vi "test Nested-Caller Two Last Acks.vi"(8 "error in (no error)":errorcluster, 11 "TestCase in":refnum<class "Test TCP Nested-Caller Two Last Acks.lvclass">) -> (0 "error out":errorcluster, 3 "TestCase out":refnum<class "Test TCP Nested-Caller Two Last Acks.lvclass">)   [LabVIEW 2020, in "Test TCP Nested-Caller Two Last Acks.lvclass"]
uses:
  Test TCP Nested-Caller Two Last Acks.lvclass
  <vilib>/addons/_JKI Toolkits/VI Tester/TestCase.llb/TestCase.lvclass
  <vilib>/ActorFramework/Message Queue/Message Queue.lvclass
  <vilib>/ActorFramework/LastAck/Last Ack.lvclass
  <vilib>/ActorFramework/Message Dequeuer/Message Dequeuer.lvclass
  Support/Caller Test Harness/Caller Test Harness Messages/Write String Data Msg/Write String Data Msg.lvclass
  Support/Caller Test Harness/Caller Test Harness/Caller Test Harness.lvclass
  Source/Nested Endpoint/Nested Endpoint/Nested Endpoint.lvclass
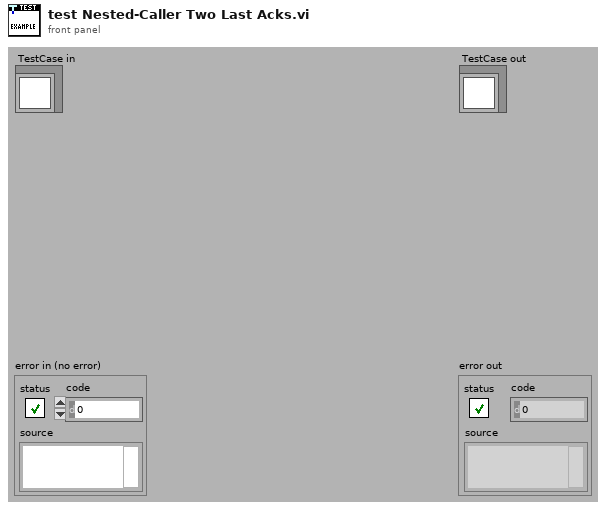
[diagram p1: front panel]
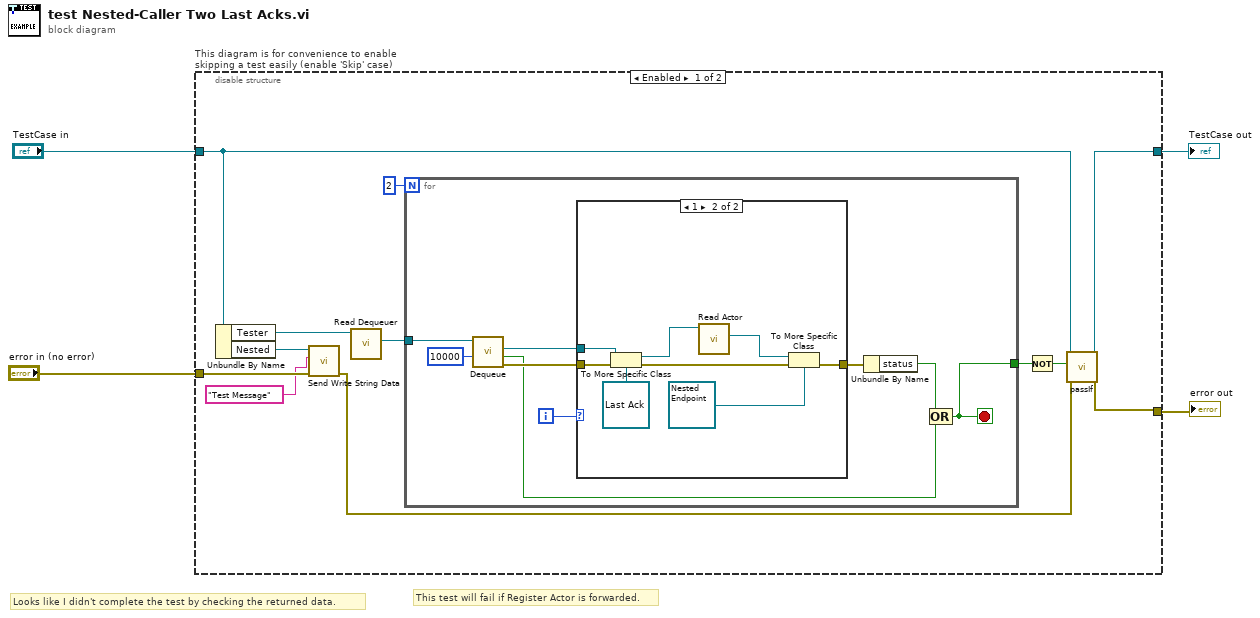
[diagram p0: block diagram]
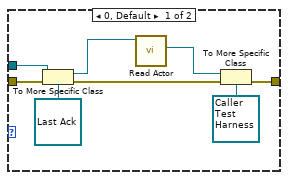
[diagram p2: hidden frame]
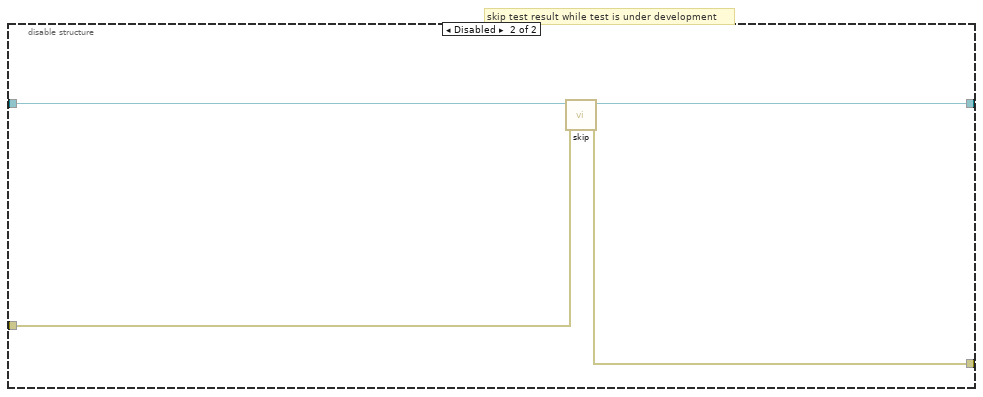
[diagram p3: hidden frame]
diagram:
  # "Looks like I didn't complete the test by checking the returned data."
  # "This test will fail if Register Actor is forwarded."
  n1 = disable-structure "This diagram is for convenience to enable skipping a test easily (enable 'Skip' case)" shown="Enabled" {
    disable-tunnel: "TestCase in" -> [w14 w45]
    disable-tunnel: [w16 w43] -> w1
    disable-tunnel: [w15 w44] -> w3
    disable-tunnel: "error in (no error)" -> [w9 w42]
    frame Enabled {
      n2 = Unbundle By Name(w14) -> ("Tester"=w13:refnum<class "Message Queue.lvclass">, "Nested"=w10:refnum<class "Message Enqueuer.lvclass">)
      n3 = call "Send Write String Data.vi"("error in (no error)"=w9, "String Data"="Test Message", "Message Enqueuer"=w10) -> ("error out"=w6:errorcluster)  [unwired: 7 in, 1 out]
      n4 = call <vilib>:"Read Dequeuer.vi"("Message Queue"=w13) -> ("Message Dequeuer"=w12:refnum<class "Message Dequeuer.lvclass">)  [unwired: 10 in]
      n5 = for {
        N: 2 -> [_]
        tunnel: w12 -> [w25]
        tunnel: [w18] -> w11
        i -> [w21]
        stop <- w18 stop-if-true
        n6 = call <vilib>:"Dequeue.vi"("timeout in ms (-1)"=10000, "Message Dequeuer in"=w25) -> ("error out"=w23:errorcluster, "timed out?"=w22:bool, "Message"=w17:refnum<class "Message.lvclass">)  [unwired: 5 in, 2 out]
        n7 = case shown="1" w21 {
          tunnel: w23 -> [w33 w41]
          tunnel: w17 -> [w31 w39]
          tunnel: [w28 w36] -> w20
          frame 0, Default {
            n8 = To More Specific Class(target class=refnum<class "Last Ack.lvclass"> refnum ("Last Ack"), reference=w31, error in=w33) -> (specific class reference=w27:refnum<class "Last Ack.lvclass">, error out=w30:errorcluster)
            n9 = call <vilib>:"Read Actor.vi"("Last Ack"=w27) -> ("Actor"=w26:refnum<class "Actor.lvclass">)  [unwired: 10 in]
            n10 = To More Specific Class(target class=refnum<class "Caller Test Harness.lvclass"> refnum ("Caller Test Harness.lvlib:Caller Test Harness.lvclass"), reference=w26, error in=w30) -> (error out=w28:errorcluster)  [unwired: 1 out]
          }
          frame 1 {
            n11 = To More Specific Class(target class=refnum<class "Last Ack.lvclass"> refnum ("Last Ack"), reference=w39, error in=w41) -> (specific class reference=w37:refnum<class "Last Ack.lvclass">, error out=w38:errorcluster)
            n12 = call <vilib>:"Read Actor.vi"("Last Ack"=w37) -> ("Actor"=w34:refnum<class "Actor.lvclass">)  [unwired: 10 in]
            n13 = To More Specific Class(target class=refnum<class "Nested Endpoint.lvclass"> refnum ("Nested Endpoint.lvlib:Nested Endpoint.lvclass"), reference=w34, error in=w38) -> (error out=w36:errorcluster)  [unwired: 1 out]
          }
        }
        n14 = Unbundle By Name(w20) -> ("status"=w19:bool)
        n15 = Compound Arithmetic op=OR(w19, w22) -> (w18:bool)
      }
      n16 = Not(x=w11) -> (.not. x?=w5:bool)
      n17 = call-dynamic "passIf.vi"("error in (no error)"=w6, "pass"=w5, "TestCase in"=w14) -> ("error out"=w15:errorcluster, "TestCase out"=w16:refnum<class "Test TCP Nested-Caller Two Last Acks.lvclass">)  [unwired: 7 in]
    }
    frame Disabled {
      # "skip test result while test is under development"
      n18 = call <vilib>:"skip.vi"("error in (no error)"=w42, "TestCase in"=w45) -> ("error out"=w44:errorcluster, "TestCase out"=w43:refnum<class "Test TCP Nested-Caller Two Last Acks.lvclass">)  [unwired: 8 in]
    }
  }
  "error out" <- w3
  "TestCase out" <- w1
